vi "epx_Vector.Type Write.vi"(4 "error in (no error)":errorcluster, 5 "Value":T2, 6 "Container State":T3, 7 "Display State In":T1={"BGColor"=16448250, "FGColor"=0, "GridColor"=9868950, "Number of Polar Grids"=12, "Number of Circle Grids"=4, "Vector.Active"=0, "Vectors.Properties"=[], "Height"=0, "Width"=0} {"Number of Circle Grids" min=1 max=100 step=1; "Number of Polar Grids" min=1 max=100 step=1}) -> (0 "error out":errorcluster, 3 "Display State Out":T1={"BGColor"=16448250, "FGColor"=0, "GridColor"=9868950, "Number of Polar Grids"=12, "Number of Circle Grids"=4, "Vector.Active"=0, "Vectors.Properties"=[], "Height"=0, "Width"=0} {"Number of Circle Grids" min=1 max=100 step=1; "Number of Polar Grids" min=1 max=100 step=1})   [LabVIEW 2011, in "NI_EP_Basic.lvlib" / "EPX Vector Diagram.xctl"]
uses:
  <vilib>/addons/Electrical Power/Basic/Controls/Vector Diagram/EPX Vector Diagram.xctl
  <vilib>/_xctls/Container State.ctl
  <vilib>/addons/Electrical Power/Basic/Controls/Vector Diagram/SubVIs/epx_Vector Type.ctl
  <vilib>/addons/Electrical Power/Basic/Controls/Vector Diagram/Abilities/epx_Vector Diagram State.ctl
  <vilib>/_xctls/XControlSupport.lvlib
  <vilib>/addons/Electrical Power/Basic/NI_EP_Basic.lvlib
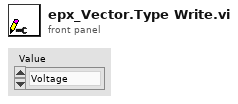
[diagram p1: front panel]
types:
  T1 = typedef "NI_EP_Basic.lvlib/EPX Vector Diagram.xctl/epx_Vector Diagram State.ctl" = cluster{"BGColor":u32, "FGColor":u32, "GridColor":u32, "Number of Polar Grids":i32, "Number of Circle Grids":i32, "Vector.Active":i32, "Vectors.Properties":cluster{"Vector.Type":T2, "Vector.Color":u32, "Vector.Width":u8}[], "Height":u32, "Width":u32}
  T2 = typedef "NI_EP_Basic.lvlib/epx_Vector Type.ctl" = enum16{"Voltage", "Current"}
  T3 = typedef "XControlSupport.lvlib/Container State.ctl" = cluster{"Indicator?":bool, "Run Mode?":bool, " Refnum":refnum<vi>}
  T4 = cluster{"Vector.Type":T2, "Vector.Color":u32, "Vector.Width":u8}[]
  T5 = cluster{"Vector.Type":T2, "Vector.Color":u32, "Vector.Width":u8}
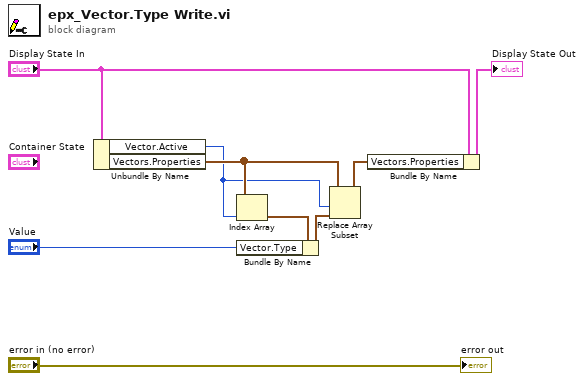
[diagram p0: block diagram]
diagram:
  n1 = Unbundle By Name("Display State In") -> ("Vector.Active"=w6:i32, "Vectors.Properties"=w7:T4)
  n2 = Index Array(array=w7, index=w6) -> (element=w8:T5)
  n3 = Bundle By Name(cluster=w8, "Vector.Type"="Value") -> (w4:T5)
  n4 = Replace Array Subset(array=w7, new element=w4, index=w6) -> (w5:T4)
  n5 = Bundle By Name(cluster="Display State In", "Vectors.Properties"=w5) -> (→"Display State Out":T1)
  "error out" <- "error in (no error)"
